vi "test_NI.vi"() -> ()   [LabVIEW 2020]
uses:
  <vilib>/Platform/TimedLoop/XDataNode/wakeup.ctl
  <vilib>/Platform/TimedLoop/XDataNode/XDNodeRunTimeDep.lvlib
  <vilib>/Platform/TimedLoop/XDataNode/nitl_modes.ctl
  <vilib>/Platform/TimedLoop/XDataNode/timing_clust.ctl
  <vilib>/Platform/TimedLoop/XDataNode/XDataNode.xnode
panel:
  in  "删除路径":path
  in  "创建文件夹路径":path
  in  "file path (use dialog)":path=path "C:/data_xyx_LuGre.bin"
  in  "save data":bool=TRUE
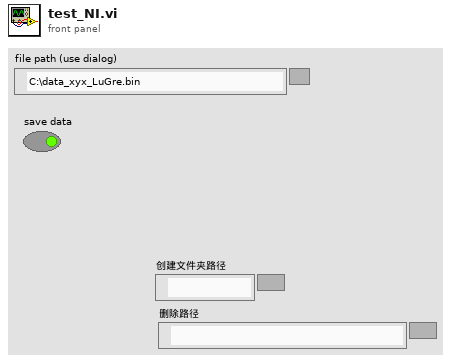
[diagram p1: front panel]
types:
  T1 = enum16{"open", "replace", "create", "open or create", "replace or create", "replace or create with confirmation"}
  T2 = typedef "XDNodeRunTimeDep.lvlib/timing_clust.ctl" = cluster{"Expected End [f-1]":u64, "Actual End [f-1]":u64, "Finished Late? [f-1]":bool, "Expected End [i-1]":u64, "Actual End [i-1]":u64, "Finished Late? [i-1]":bool, "Expected Start [i]":u64, "Actual Start [i]":u64, "Expected Start [f]":u64, "Actual Start [f]":u64, "Source Name":string, "Structure Name":string, "Period":i64, "Deadline":i64, "Offset":i64, "Start":i64, "Priority":i32, "Timeout":i32, "Mode":T3, "Wakeup Reason":T4, "Error":errorcluster, "Source Type":string, "Secondary Source Type":string, "Global End Time":u64, "Global Start Time":u64, "Frame Duration":u64, "Iteration Duration":u64, "Assigned CPU":i32, "I/O Scan Engine Mode":u32}
  T3 = typedef "XDNodeRunTimeDep.lvlib/nitl_modes.ctl" = enum32{"No Change", "Process missed periods, maintain original phase", "Discard missed periods, maintain original phase", "Process missed periods, ignore original phase", "Discard missed periods, ignore original phase"}
  T4 = typedef "XDNodeRunTimeDep.lvlib/wakeup.ctl" = enum32{"Normal", "Aborted", "Asynchronous wakeup", "Timing source error", "Timed loop error", "Timeout"}
  T5 = enum16{"big-endian, network order", "native, host order", "little-endian"}
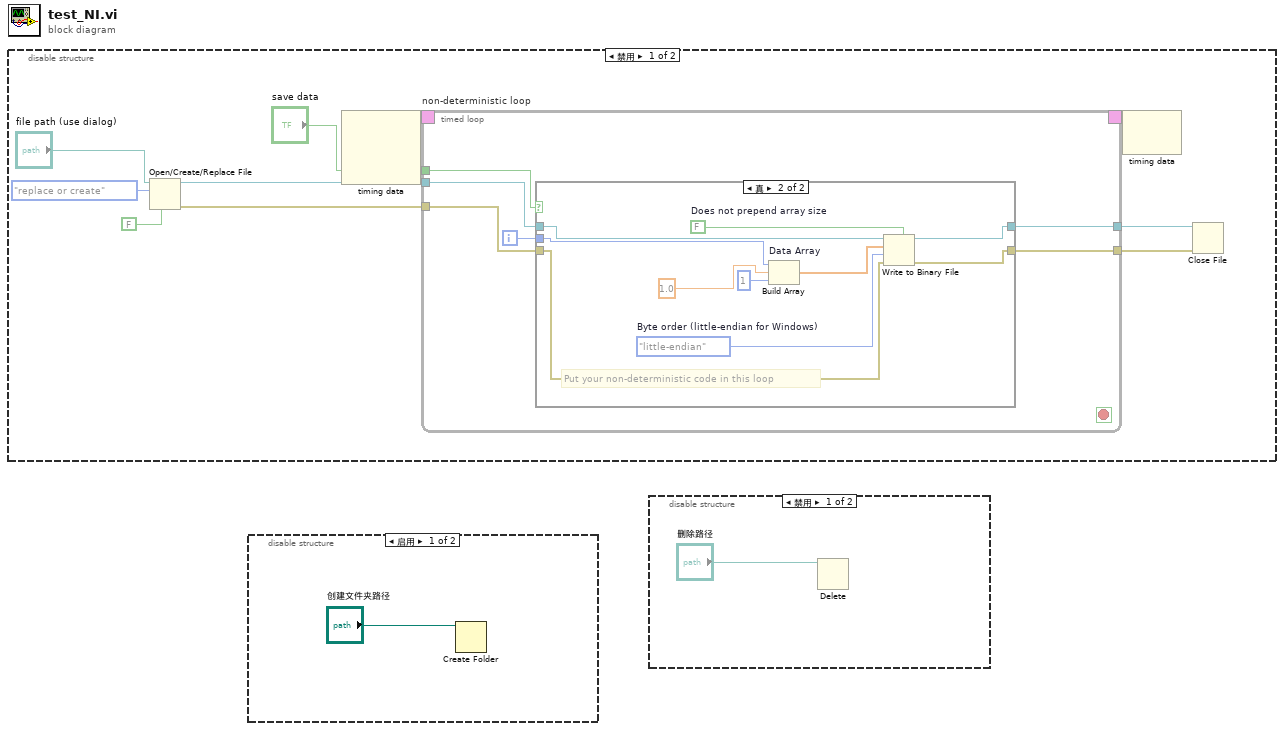
[diagram p0: block diagram]
diagram:
  n1 = disable-structure shown="禁用" {
    frame Disabled {
      n2 = Open/Create/Replace File(file path (use dialog)="file path (use dialog)", operation (0:open)=T1."replace or create", disable buffering (F)=FALSE) -> (refnum out=w6:refnum<file>, error out=w5:errorcluster)  [unwired: 3 in, 1 out]
      n3 = node-c288 ("Input Node")() -> (w10:T2)  [unwired: 3 in]
      n4 = timed-loop "non-deterministic loop" {
        timing: w10 -> [_]
        timing-out: [_] -> w9
        tunnel: [w16] -> w3
        tunnel: w5 -> [w15]
        tunnel: [w14] -> w4
        tunnel: "save data" -> [w13]
        tunnel: w6 -> [w12]
        i -> [w11]
        stop <- _ stop-if-true
        n5 = case shown="真" w13 {
          tunnel: [w17 w28] -> w16
          tunnel: w12 -> [w18 w27]
          tunnel: w15 -> [w17 w26]
          tunnel: [w18 w23] -> w14
          tunnel: w11 -> [_ w21]
          frame False {
          }
          frame True {
            w24 = FALSE  # Does not prepend array size
            w25 = T5."little-endian"  # Byte order (little-endian for Windows)
            # "Put your non-deterministic code in this loop"
            n6 = Build Array "Data Array"(w21, 1.0, 1) -> (w22:dbl[])
            n7 = Write to Binary File(file (use dialog)=w27, data=w22, error in=w26, 5:w24, 9:w25) -> (refnum out=w23:refnum<file>, error out=w28:errorcluster)  [unwired: 1 in, 1 out]
          }
        }
      }
      n8 = node-c288 ("Output Node")(w9) -> ()  [unwired: 1 out]
      n9 = Close File(refnum=w4, error in=w3) -> ()  [unwired: 2 out]
    }
    frame Enabled {
    }
  }
  n10 = disable-structure shown="启用" {
    frame Enabled {
      n11 = Create Folder(path (use dialog)="创建文件夹路径") -> ()  [unwired: 2 in, 3 out]
    }
    frame Disabled {
    }
  }
  n12 = disable-structure shown="禁用" {
    frame Disabled {
      n13 = Delete(path (use dialog)="删除路径") -> ()  [unwired: 4 in, 3 out]
    }
    frame Enabled {
    }
  }
